vi "Configure POWER DOWN.vi"(7 "All Channels (F)":bool, 8 "error in (no error)":errorcluster, 9 "Power down (KILL)":string(combo)="KILL", 10 "Channel (0)":u8, 11 "BoardHandle":T1) -> (0 "error out":errorcluster, 3 "BoardHandle out":T1)   [LabVIEW 2009, in "CAEN PSM.lvlib"]
doc: "This function allows to configure Power Down mode."
uses:
  <instrlib>/CAEN PSM/CAEN PSM.lvlib
  <instrlib>/CAEN PSM/Private/BoardHandle.ctl
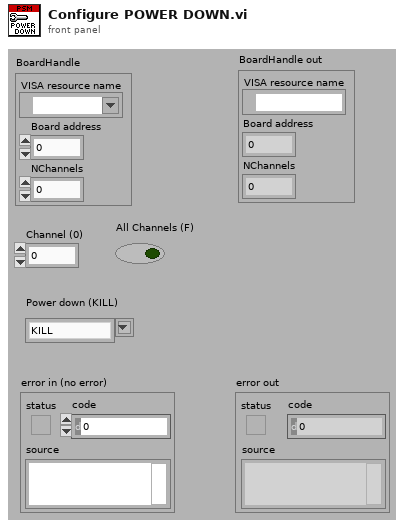
[diagram p1: front panel]
types:
  T1 = typedef "CAEN PSM.lvlib/BoardHandle.ctl" = cluster{"VISA resource name":refnum<visa-resource-name>, "Board address":u8, "NChannels":u8}
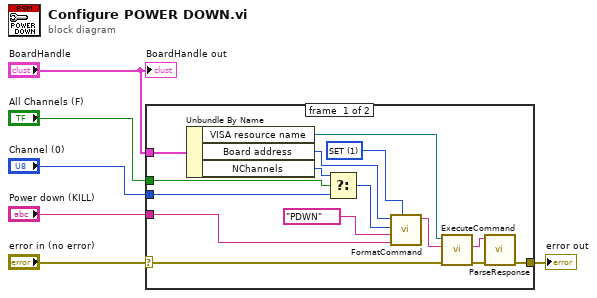
[diagram p0: block diagram]
diagram:
  n1 = case shown="No Error" "error in (no error)" {
    selector: "error in (no error)" -> [w9 w22]
    tunnel: "Power down (KILL)" -> [w7 _]
    tunnel: "All Channels (F)" -> [w19 _]
    tunnel: "Channel (0)" -> [w17 _]
    tunnel: [w12 w22] -> w3
    tunnel: "BoardHandle" -> [w10 _]
    frame #0 {
      w20 = u8 1 items=["MON", "SET"] ("CMD")
      n2 = Unbundle By Name(w10) -> ("VISA resource name"=w15:refnum<visa-resource-name>, "Board address"=w21:u8, "NChannels"=w18:u8)
      n3 = Select(t=w18, s=w19, f=w17) -> (s? t:f=w16:u8)
      n4 = call <instrlib>:"FormatCommand.vi"("CMD (MON)"=w20, "VAL"=w7, "PAR"="PDWN", "CH"=w16, "BD (0)"=w21) -> ("cmd"=w14:string)  [unwired: 6 in]
      n5 = call <instrlib>:"ExecuteCommand.vi"("error in (no error)"=w9, "Command"=w14, "VISA resource name"=w15) -> ("error out"=w13:errorcluster, "Response"=w11:string)  [unwired: 6 in, 1 out]
      n6 = call <instrlib>:"ParseResponse.vi"("error in (no error)"=w13, "Response"=w11) -> ("error out"=w12:errorcluster)  [unwired: 6 in, 3 out]
    }
    frame #1 {
    }
  }
  "error out" <- w3
  "BoardHandle out" <- "BoardHandle"
